vi "GetProperties.vi"(8 "error in":errorcluster, 11 "SlideScale in":refnum<class "SlideScale.lvclass">) -> (0 "error out":errorcluster, 3 "SlideScale out":refnum<class "SlideScale.lvclass">)   [LabVIEW 2014, in "SlideScale.lvclass"]
uses:
  SlideScale.lvclass
  SlideScale.lvclass/SlideScale.ctl
  Scale/Scale.lvclass
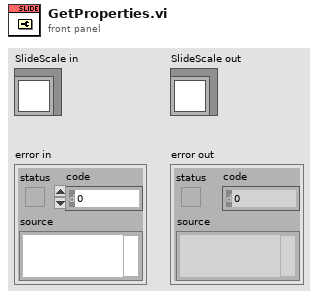
[diagram p1: front panel]
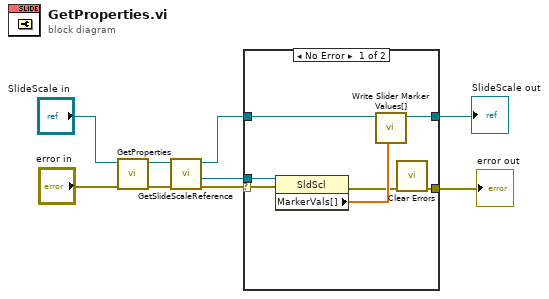
[diagram p0: block diagram]
diagram:
  n1 = call-parent "GetProperties.vi"("error in"="error in", "Scale in"="SlideScale in") -> ("error out"=w6:errorcluster, "Scale out"=w7:refnum<class "SlideScale.lvclass">)  [unwired: 8 in]
  n2 = call "GetSlideScaleReference.vi"("error in"=w6, "RotaryColorScale in"=w7) -> ("error out"=w5:errorcluster, "slide scale reference"=w4:refnum<vi>, "RotaryColorScale out"=w3:refnum<class "SlideScale.lvclass">)  [unwired: 7 in]
  n3 = case shown="No Error" w5 {
    selector: w5 -> [w16 w17]
    tunnel: w4 -> [w15 _]
    tunnel: w3 -> [w14 w18]
    tunnel: [w12 w18] -> w2
    tunnel: [w10 w17] -> w1
    frame No Error {
      n4 = property class="SldScl"(reference=w15, error in=w16) -> (error out=w11:errorcluster, "MarkerVals[]"=w13:dbl[])  [unwired: 1 out]
      n5 = call "Write Slider Marker Values[].vi"("Marker Values[]"=w13, "SlideScale in"=w14) -> ("SlideScale out"=w12:refnum<class "SlideScale.lvclass">)  [unwired: 7 in]
      n6 = call <vilib>:"Clear Errors.vi"("error in (no error)"=w11) -> ("error out"=w10:errorcluster)  [unwired: 5 in, 1 out]
    }
    frame Error {
    }
  }
  "error out" <- w1
  "SlideScale out" <- w2
